vi "Add Device.vi"(8 "error in (no error)":errorcluster, 11 "Node Ptr":u64 format="%.0x") -> (0 "error out":errorcluster)   [LabVIEW 2019, in "J1939 Addon System Explorer.lvlib"]
uses:
  J1939 Addon System Explorer.lvlib
  Addon Shared/SubVIs/Constants.vi
  Addon Shared/J1939 Addon Shared.lvlib
  <vilib>/NI VeriStand/Custom Device API/Custom Device API.lvlib
panel:
  in  "Tag":string
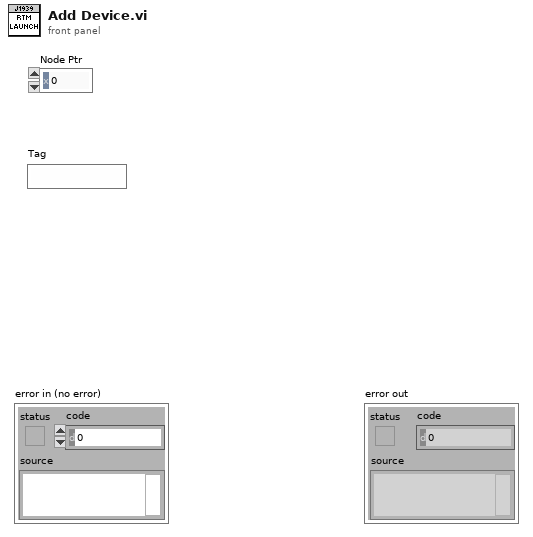
[diagram p1: front panel]
types:
  T1 = typedef "J1939 Addon Shared.lvlib/Monitor Settings.ctl" = cluster{"Address":u8, "Name":u64, "Include DA":bool}
  T2 = typedef "Custom Device API.lvlib/Custom Device Item Ref.ctl" = u64
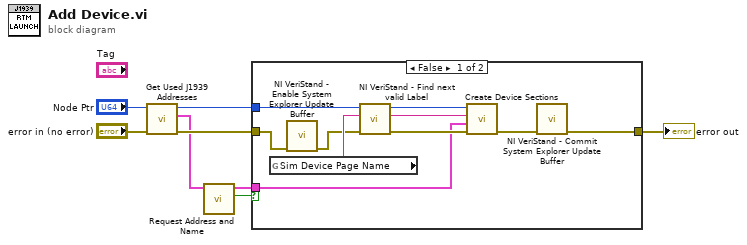
[diagram p0: block diagram]
diagram:
  n1 = call "Get Used J1939 Addresses.vi"("error in (no error)"="error in (no error)", "Node Ptr"="Node Ptr") -> ("error out"=w2:errorcluster, "Nodes"=w1:T1[], "Item Ref out"=w3:T2)  [unwired: 7 in]
  n2 = call "Request Address and Name.vi"("Nodes"=w1) -> ("Cancel out"=w7:bool, "J1939 Monitor Settings"=w6:T1)  [unwired: 9 in]
  n3 = case shown="False" w7 {
    tunnel: w3 -> [w18 _]
    tunnel: w2 -> [w12 w19]
    tunnel: [w9 w19] -> w8
    tunnel: w6 -> [w14 _]
    frame False {
      n4 = global read "Constants.vi" "Sim Device Page Name"() -> (w13:string)
      n5 = call <vilib>:"NI VeriStand - Enable System Explorer Update Buffer.vi"("error in (no error)"=w12) -> ("error out"=w11:errorcluster)  [unwired: 10 in]
      n6 = call <vilib>:"NI VeriStand - Find next valid Label.vi"("error in (no error)"=w11, "Label"=w13, "Item Ref in"=w18) -> ("error out"=w16:errorcluster, "Label out"=w15:string, "Item Ref out"=w17:T2)  [unwired: 4 in, 2 out]
      n7 = call "Create Device Sections.vi"("error in (no error)"=w16, "J1939 Monitor Settings"=w14, "Name"=w15, "Item Ref in"=w17) -> ("error out"=w10:errorcluster)  [unwired: 6 in, 1 out]
      n8 = call <vilib>:"NI VeriStand - Commit System Explorer Update Buffer.vi"("error in (no error)"=w10) -> ("error out"=w9:errorcluster)  [unwired: 10 in]
    }
    frame True {
    }
  }
  "error out" <- w8
